vi "队列堆栈（DBL）.vi"(8 "error in (no error)":errorcluster caption="错误输入（无错误）", 9 "堆栈操作":T1, 10 "堆栈长度":i32=-1, 11 "入栈元素":dbl) -> (0 "error out":errorcluster caption="错误输出", 1 "堆栈空":bool, 2 "入栈所有元素":dbl[](array[numeric]), 3 "出栈元素":dbl)   [LabVIEW 2012]
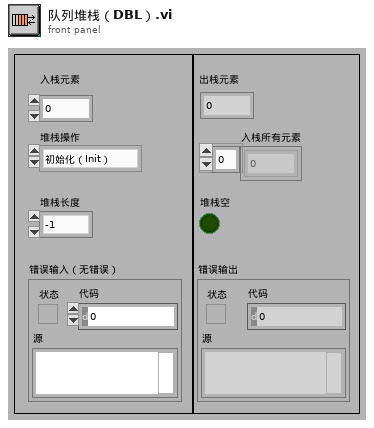
[diagram p1: front panel]
types:
  T1 = typedef "堆栈操作.ctl" = enum16{"初始化（Init）", "进栈（Push）", "出栈（Pop）", "状态（Status)", "释放"}
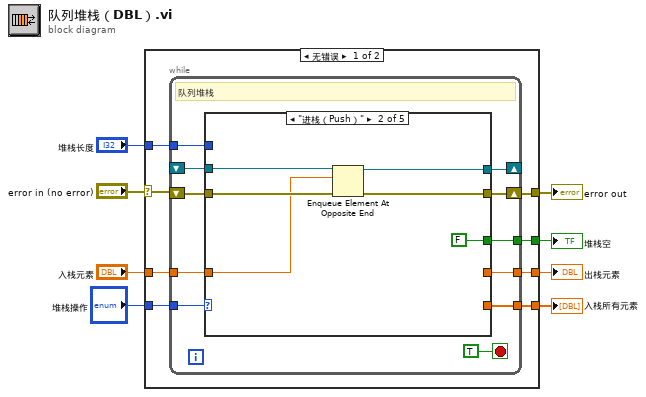
[diagram p0: block diagram]
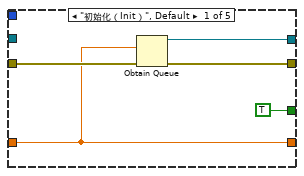
[diagram p2: hidden frame]
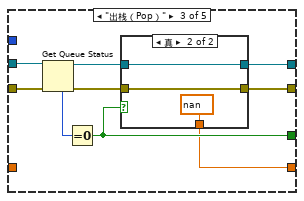
[diagram p3: hidden frame]
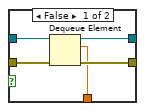
[diagram p4: hidden frame]
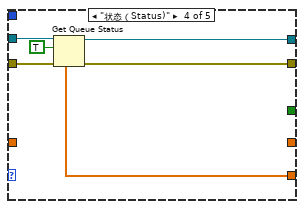
[diagram p5: hidden frame]
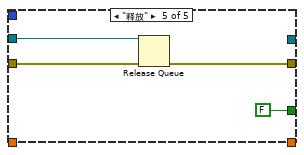
[diagram p6: hidden frame]
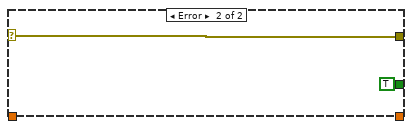
[diagram p7: hidden frame]
diagram:
  n1 = case shown="无错误" "error in (no error)" {
    selector: "error in (no error)" -> [w12 w67]
    tunnel: [w11 w67] -> w7
    tunnel: "堆栈操作" -> [w16 _]
    tunnel: "入栈元素" -> [w15 _]
    tunnel: [w14 _] -> w4
    tunnel: "堆栈长度" -> [w13 _]
    tunnel: [w10 TRUE] -> w2
    tunnel: [w9 _] -> w1
    frame No Error {
      n2 = while {
        tunnel: w16 -> [w27]
        tunnel: w15 -> [w26]
        tunnel: [w25] -> w14
        tunnel: w13 -> [w24]
        shift-right: [w21] -> w11
        shift-left: w12 -> [w22]
        shift-right: [w20] -> _
        shift-left: _ -> [w19]
        tunnel: [w18] -> w10
        tunnel: [w17] -> w9
        stop <- TRUE stop-if-true
        # "队列堆栈"
        n3 = case shown="\"进栈（Push）\"" w27 {
          tunnel: w26 -> [w29 w34 _ _ _]
          tunnel: [w29 _ w39 _ _] -> w25
          tunnel: w24 -> [_ _ _ _ _]
          tunnel: w22 -> [w32 w38 w47 w60 w65]
          tunnel: [w31 w37 w40 w57 w64] -> w21
          tunnel: [w30 w35 w42 w58 _] -> w20
          tunnel: w19 -> [_ w36 w46 w61 w63]
          tunnel: [TRUE FALSE w44 _ FALSE] -> w18
          tunnel: [_ _ _ w56 _] -> w17
          frame "初始化（Init）", Default {
            n4 = Obtain Queue(element data type=w29, error in (no error)=w32) -> (queue out=w30:refnum<queue>, error out=w31:errorcluster)  [unwired: 3 in, 1 out]
          }
          frame "进栈（Push）" {
            n5 = Enqueue Element At Opposite End(queue=w36, element=w34, error in (no error)=w38) -> (queue out=w35:refnum<queue>, error out=w37:errorcluster)  [unwired: 1 in, 1 out]
          }
          frame "出栈（Pop）" {
            n6 = Get Queue Status(queue=w46, error in (no error)=w47) -> (queue out=w43:refnum<queue>, error out=w41:errorcluster, # elements in queue=w45:i32)  [unwired: 1 in, 5 out]
            n7 = Equal To 0?(x=w45) -> (x = 0?=w44:bool)
            n8 = case shown="真" w44 {
              tunnel: w43 -> [w52 w55]
              tunnel: [w51 w55] -> w42
              tunnel: w41 -> [w50 w54]
              tunnel: [w49 w54] -> w40
              tunnel: [w48 nan ("入栈元素(CDB)")] -> w39
              frame False {
                n9 = Dequeue Element(queue=w52, error in (no error)=w50) -> (queue out=w51:refnum<queue>, element=w48:dbl, error out=w49:errorcluster)  [unwired: 1 in, 1 out]
              }
              frame True {
              }
            }
          }
          frame "状态（Status)" {
            n10 = Get Queue Status(queue=w61, return elements? (F)=TRUE ("返回元素？(F)"), error in (no error)=w60) -> (queue out=w58:refnum<queue>, error out=w57:errorcluster, elements=w56:dbl[])  [unwired: 5 out]
          }
          frame "释放" {
            n11 = Release Queue(queue=w63, error in (no error)=w65) -> (error out=w64:errorcluster)  [unwired: 1 in, 2 out]
          }
        }
      }
    }
    frame Error {
    }
  }
  "error out" <- w7
  "出栈元素" <- w4
  "堆栈空" <- w2
  "入栈所有元素" <- w1
